vi "Error Query.vi"(8 "error in (no error)":errorcluster, 11 "VISA resource name":refnum<visa-resource-name>) -> (0 "error out":errorcluster, 3 "VISA resource name out":refnum<visa-resource-name>)   [LabVIEW 2019, in "BK Precision 1823A.lvlib"]
doc: "Queries the instrument for any errors in the instrument's error queue. It will continue to read errors until all errors have been read from the instrument. Any errors will be returned in the Error Out cluster.\n\nNote:\nThis VI is called automatically by most driver VIs so it is not usually necessary to call this in an application."
uses:
  BK Precision 1823A.lvlib
panel:
  # "(c) 2009 B&K PRECISION CORPORATION.  ALL RIGHTS RESERVED."
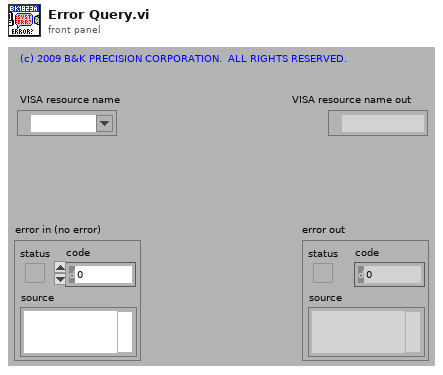
[diagram p1: front panel]
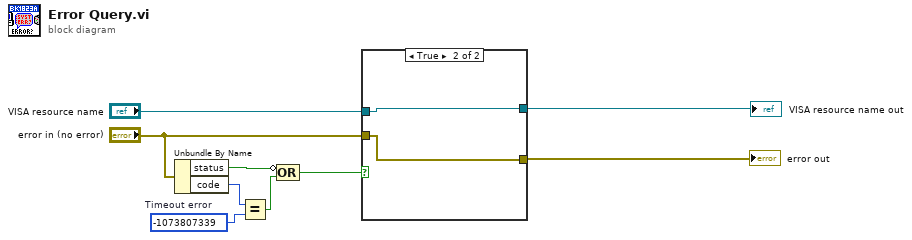
[diagram p0: block diagram]
diagram:
  w5 = -1073807339  # Timeout error
  n1 = Unbundle By Name("error in (no error)") -> ("status"=w6:bool, "code"=w3:i32)
  n2 = Equal?(x=w3, y=w5) -> (x = y?=w4:bool)
  n3 = Compound Arithmetic op=OR(invert w6, w4) -> (w2:bool)
  n4 = case shown="True" w2 {
    tunnel: [w11 w13] -> w1
    tunnel: "VISA resource name" -> [w11 w13]
    tunnel: "error in (no error)" -> [w10 w12]
    tunnel: [w10 w12] -> w8
    frame False {
      (unwired) i32[] []
      (unwired) ""
    }
    frame True {
    }
  }
  "VISA resource name out" <- w1
  "error out" <- w8
